vi "MindwaveCmpChksum.vi"(4 "error in (no error) input":errorcluster, 6 "[CHECKSUM] - CALCULATED":u8 format="%x", 7 "VISA resource name input":refnum<visa-resource-name>) -> (0 "error out":errorcluster, 2 "canParseData?":bool, 3 "VISA resource name out":refnum<visa-resource-name>)   [LabVIEW 2011, in "Neurosky.lvlib"]
uses:
  Users/Isaias/Documents/GitHub/Neurosky/Neurosky.lvlib
panel:
  out "[CHECKSUM] - MINDWAVE":u8 format="%x"
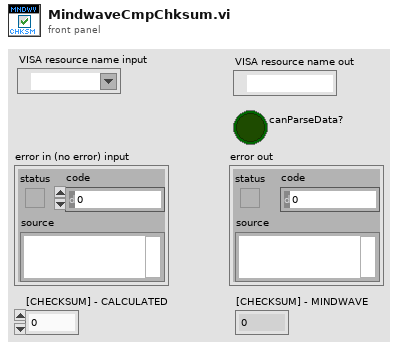
[diagram p1: front panel]
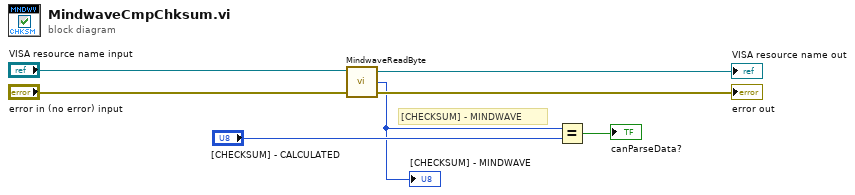
[diagram p0: block diagram]
diagram:
  # "[CHECKSUM] - MINDWAVE"
  n1 = call <userlib>:"MindwaveReadByte.vi"("error in (no error) input"="error in (no error) input", "VISA resource name input"="VISA resource name input") -> ("error out"=→"error out":errorcluster, "byte"=w2:u8, "VISA resource name out"=→"VISA resource name out":refnum<visa-resource-name>)  [unwired: 2 in]
  "[CHECKSUM] - MINDWAVE" <- w2
  n2 = Equal?(x=w2, y="[CHECKSUM] - CALCULATED") -> (x = y?=→"canParseData?":bool)
